vi "Sour_Meas_Instrument.vi"(0 "Command":string="SOURce:VOLTage:DC 10", 11 "Error_In":errorcluster) -> (4 "Responce":dbl, 6 "Action":string, 8 "Parameter":string, 15 "Error_Out":errorcluster)   [LabVIEW 2021]
doc: "This VI SOURce and MEASure the data with the command provided.\nSOURce- Storing the data into the INI file.\nMEASure - Retrieving the data from the INI file."
uses:
  <vilib>/Utility/config.llb/NI_LVConfig.lvlib
  <vilib>/Utility/config.llb/Read Key (Double).vi
  <vilib>/numeric/Random Number (Range) DBL.vi
  <vilib>/Utility/config.llb/Write Key (Double).vi
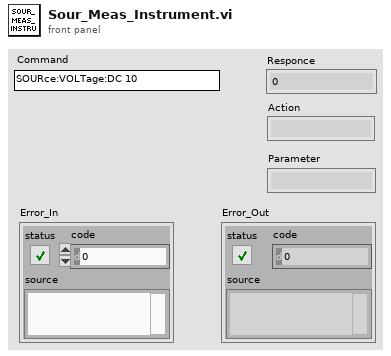
[diagram p1: front panel]
types:
  T1 = typedef "NI_LVConfig.lvlib/Config Data RefNum.ctl" = refnum<k1>
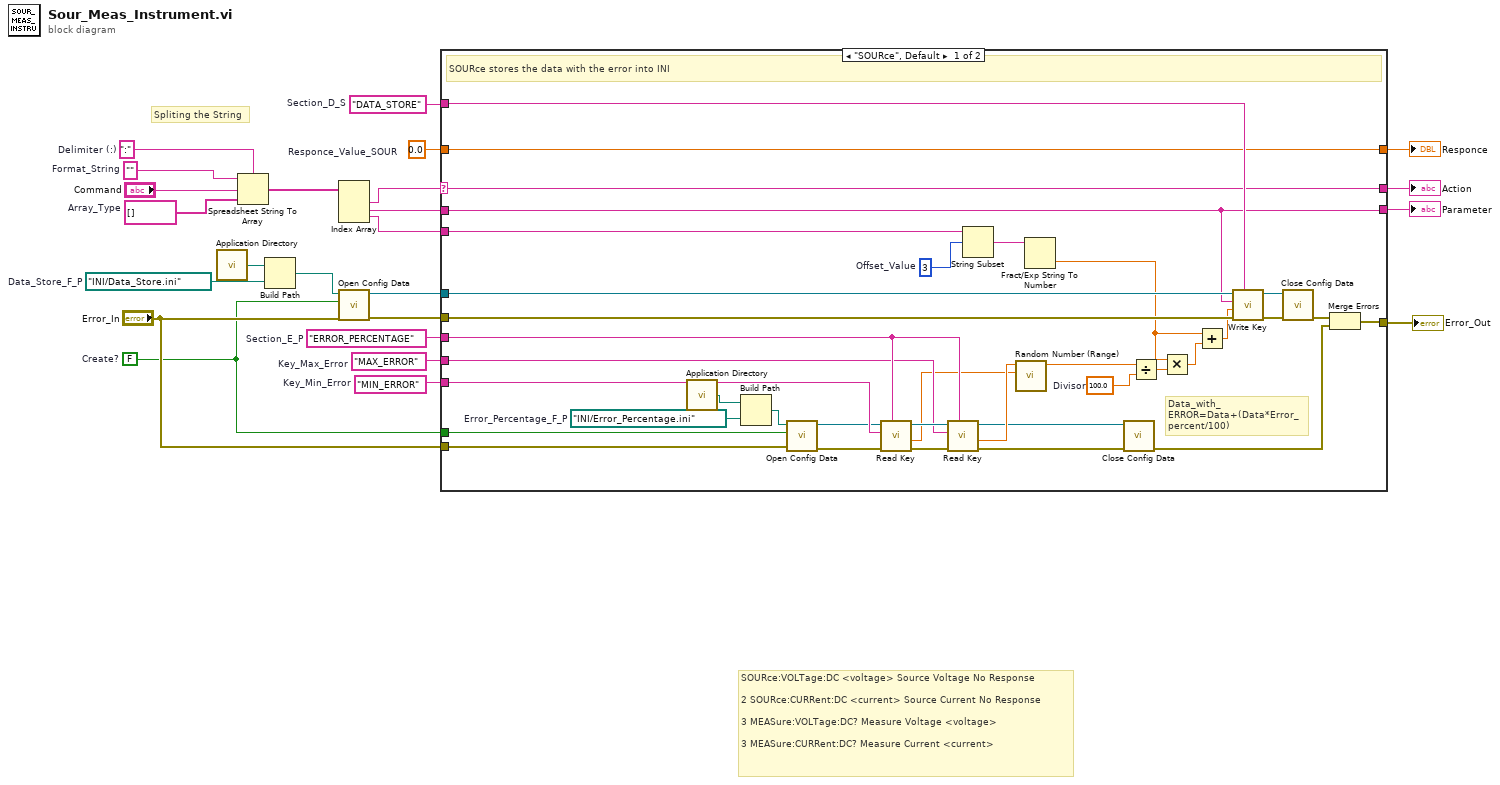
[diagram p0: block diagram]
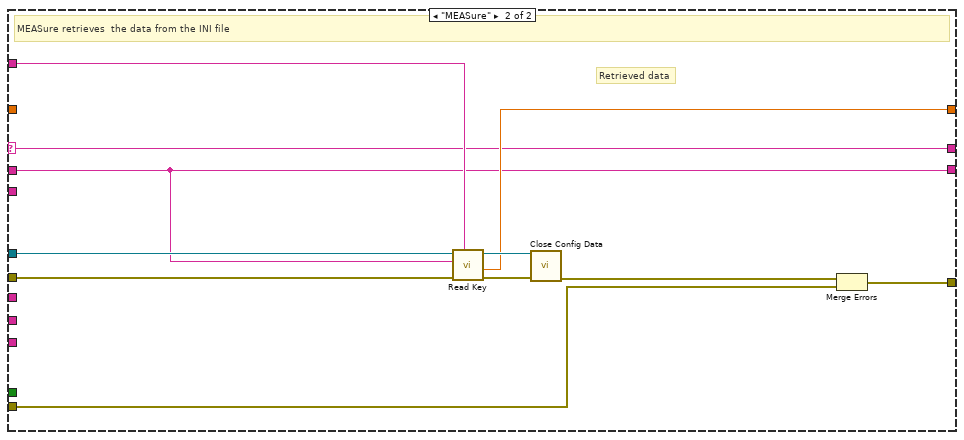
[diagram p2: hidden frame]
diagram:
  w7 = 0.0  # Responce_Value_SOUR
  w11 = "MIN_ERROR"  # Key_Min_Error
  w12 = "MAX_ERROR"  # Key_Max_Error
  w13 = "ERROR_PERCENTAGE"  # Section_E_P
  w4 = FALSE  # Create?
  w14 = "DATA_STORE"  # Section_D_S
  w1 = path "INI/Data_Store.ini"  # Data_Store_F_P
  w21 = ""  # Format_String
  w24 = string[] []  # Array_Type
  w22 = ":"  # Delimiter (:)
  # "Spliting the String"
  # "SOURce:VOLTage:DC <voltage> Source Voltage No Response\n\n2 SOURce:CURRent:DC <current> Source Current No Response\n\n3 MEASure:VOLTage:DC? Measure Voltage <voltage>\n\n3 MEASure:CURRent:DC? Measure Current <current>"
  n1 = call <vilib>:"Application Directory.vi"() -> ("Application Directory"=w2:path)
  n2 = Spreadsheet String To Array(delimiter (Tab)=w22, format string=w21, spreadsheet string="Command", array type (2D Dbl)=w24) -> (array=w19:string[])
  n3 = Build Path(base path=w2, name or relative path=w1) -> (appended path=w3:path)
  n4 = Index Array(array=w19) -> (element #1=w20:string, element #2=w18:string, element #3=w17:string)  [unwired: 3 in]
  n5 = call <vilib>:"Open Config Data.vi"("error in (no error)"="Error_In", "create file if necessary (T)"=w4, "configuration file path"=w3) -> ("error out"=w16:errorcluster, "refnum"=w15:T1)  [unwired: 6 in, 1 out]
  n6 = case shown="\"SOURce\", Default" w20 {
    selector: w20 -> [w41 w65]
    tunnel: w18 -> [w40 w64]
    tunnel: w17 -> [w32 _]
    tunnel: w16 -> [w59 w69]
    tunnel: w15 -> [w60 w70]
    tunnel: w14 -> [w52 w71]
    tunnel: [w39 w66] -> w6
    tunnel: "Error_In" -> [w28 w61]
    tunnel: w13 -> [w49 _]
    tunnel: w12 -> [w47 _]
    tunnel: w11 -> [w48 _]
    tunnel: [w38 w62] -> w10
    tunnel: [w41 w65] -> w9
    tunnel: [w40 w64] -> w8
    tunnel: w7 -> [w39 _]
    tunnel: w4 -> [w31 _]
    frame "SOURce", Default {
      w27 = path "INI/Error_Percentage.ini"  # Error_Percentage_F_P
      w43 = 100.0  # Divisor
      w33 = 3  # Offset_Value
      # "Data_with_ERROR=Data+(Data*Error_percent/100)"
      # "SOURce stores the data with the error into INI"
      n7 = call <vilib>:"Application Directory.vi"() -> ("Application Directory"=w26:path)
      n8 = Build Path(base path=w26, name or relative path=w27) -> (appended path=w25:path)
      n9 = call <vilib>:"Open Config Data.vi"("error in (no error)"=w28, "create file if necessary (T)"=w31, "configuration file path"=w25) -> ("error out"=w30:errorcluster, "refnum"=w29:T1)  [unwired: 6 in, 1 out]
      n10 = call-poly <vilib>:"Read Key.vi"("section"=w49, "error in (no error)"=w30, "key"=w48, "refnum"=w29) -> ("error out"=w50:errorcluster, "value"=w45:dbl, "refnum out"=w51:T1)  [unwired: 4 in, 1 out]
      n11 = call-poly <vilib>:"Read Key.vi"("section"=w49, "error in (no error)"=w50, "key"=w47, "refnum"=w51) -> ("error out"=w36:errorcluster, "value"=w46:dbl, "refnum out"=w37:T1)  [unwired: 4 in, 1 out]
      n12 = String Subset(string=w32, offset (0)=w33) -> (substring=w34:string)  [unwired: 1 in]
      n13 = call-poly <vilib>:"Random Number (Range).vi"("lower bound (0)"=w45, "upper bound (100)"=w46) -> ("number"=w44:dbl)  [unwired: 9 in]
      n14 = Fract/Exp String To Number(string=w34) -> (number=w56:dbl)  [unwired: 3 in, 1 out]
      n15 = call <vilib>:"Close Config Data.vi"("error in (no error)"=w36, "refnum"=w37) -> ("error out"=w35:errorcluster)  [unwired: 8 in, 1 out]
      n16 = Divide(x=w44, y=w43) -> (x/y=w58:dbl)
      n17 = Multiply(x=w56, y=w58) -> (x*y=w57:dbl)
      n18 = Add(x=w56, y=w57) -> (x+y=w55:dbl)
      n19 = call-poly <vilib>:"Write Key.vi"("section"=w52, "error in (no error)"=w59, "value"=w55, "key"=w40, "refnum"=w60) -> ("error out"=w53:errorcluster, "refnum out"=w54:T1)  [unwired: 4 in, 1 out]
      n20 = call <vilib>:"Close Config Data.vi"("error in (no error)"=w53, "refnum"=w54) -> ("error out"=w42:errorcluster)  [unwired: 8 in, 1 out]
      n21 = Merge Errors(w42, w35) -> (w38:errorcluster)
    }
    frame "MEASure" {
      # "Retrieved data"
      # "MEASure retrieves  the data from the INI file"
      n22 = call-poly <vilib>:"Read Key.vi"("section"=w71, "error in (no error)"=w69, "key"=w64, "refnum"=w70) -> ("error out"=w67:errorcluster, "value"=w66:dbl, "refnum out"=w68:T1)  [unwired: 4 in, 1 out]
      n23 = call <vilib>:"Close Config Data.vi"("error in (no error)"=w67, "refnum"=w68) -> ("error out"=w63:errorcluster)  [unwired: 8 in, 1 out]
      n24 = Merge Errors(w63, w61) -> (w62:errorcluster)
    }
  }
  "Responce" <- w6
  "Error_Out" <- w10
  "Action" <- w9
  "Parameter" <- w8
